vi "Move If.vi"(8 "If":T2[](array[typedef]), 9 "Move":T2[](array[typedef]), 10 "1D Maze":i32[](array[numeric]), 11 "Class":refnum<class "Pinwheel.lvclass">) -> (1 "Action":T1, 2 "Direction":T2, 3 "Class":refnum<class "Pinwheel.lvclass">)   [LabVIEW 2015, in "Pinwheel.lvclass"]
uses:
  Pinwheel.lvclass
  Type Defs/Action Enum.ctl
  Type Defs/SB Type Defs.lvlib
  Type Defs/Direction Enum.ctl
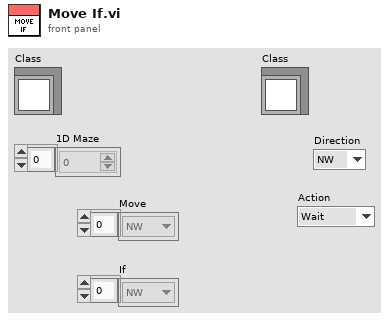
[diagram p1: front panel]
types:
  T1 = typedef "SB Type Defs.lvlib/Action Enum.ctl" = enum16{"Wait", "Move", "Attack", "Replicate"}
  T2 = typedef "SB Type Defs.lvlib/Direction Enum.ctl" = enum16{"NW", "N", "NE", "E", "SE", "S", "SW", "W"}
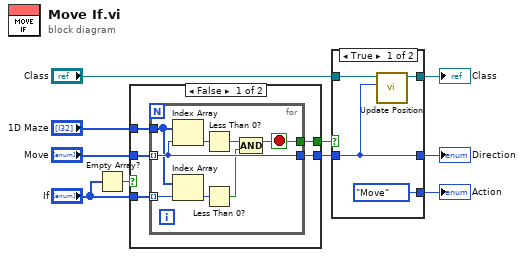
[diagram p0: block diagram]
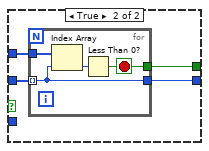
[diagram p2: hidden frame]
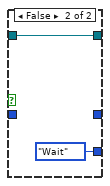
[diagram p3: hidden frame]
diagram:
  n1 = Empty Array?(array="If") -> (empty?=w1:bool)
  n2 = case shown="False" w1 {
    tunnel: "Move" -> [w15 w27]
    tunnel: [w14 w26] -> w9
    tunnel: [w13 w25] -> w8
    tunnel: "1D Maze" -> [w12 w24]
    tunnel: "If" -> [w11 _]
    frame False {
      n3 = for {
        tunnel: [w17] -> w13
        tunnel: w12 -> [w21]
        tunnel: [w22] -> w14
        tunnel: w15 -> [w22] mode=indexing
        tunnel: w11 -> [w20] mode=indexing
        stop <- w17 stop-if-true
        n4 = Index Array(array=w21, index=w22) -> (element=w23:i32)
        n5 = Index Array(array=w21, index=w20) -> (element=w19:i32)
        n6 = Less Than 0?(x=w23) -> (x < 0?=w18:bool)
        n7 = Less Than 0?(x=w19) -> (x < 0?=w16:bool)
        n8 = Compound Arithmetic op=AND(w18, w16) -> (w17:bool)
      }
    }
    frame True {
      n9 = for {
        tunnel: [w28] -> w25
        tunnel: w24 -> [w29]
        tunnel: [w30] -> w26
        tunnel: w27 -> [w30] mode=indexing
        stop <- w28 stop-if-true
        n10 = Index Array(array=w29, index=w30) -> (element=w31:i32)
        n11 = Less Than 0?(x=w31) -> (x < 0?=w28:bool)
      }
    }
  }
  n12 = case shown="True" w8 {
    tunnel: "Class" -> [w34 w36]
    tunnel: [Action_Enum."Move" ("Action") Action_Enum."Wait" ("Action")] -> w5
    tunnel: w9 -> [w33 _]
    tunnel: [w33 _] -> w6
    tunnel: [w32 w36] -> w7
    frame True {
      n13 = call "Update Position.vi"("Direction"=w33, "Class"=w34) -> ("Class"=w32:refnum<class "Pinwheel.lvclass">)  [unwired: 9 in]
    }
    frame False {
    }
  }
  "Class" <- w7
  "Direction" <- w6
  "Action" <- w5
